vi "GPS -Get Lat Lng from Address.vi"(8 "error in (no error)":errorcluster, 11 "keywords":string="Calgary, Alberta, CANADA") -> (0 "error out":errorcluster, 1 "Lng":dbl, 3 "Lat":dbl, 5 "LngStrg":string, 7 "LatStrg":string)   [LabVIEW 2019]
uses:
  \\mac\Dropbox/gmap.net/GMAP.NET 8.6/data/GMap.NET.Core.dll
  data/GMap.NET.Core.dll
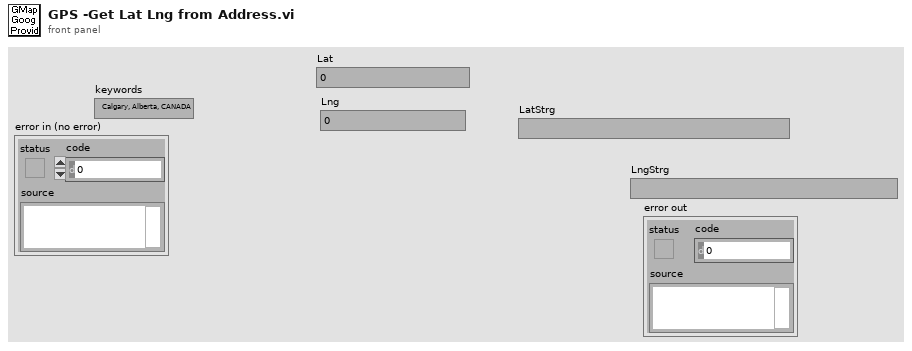
[diagram p1: front panel]
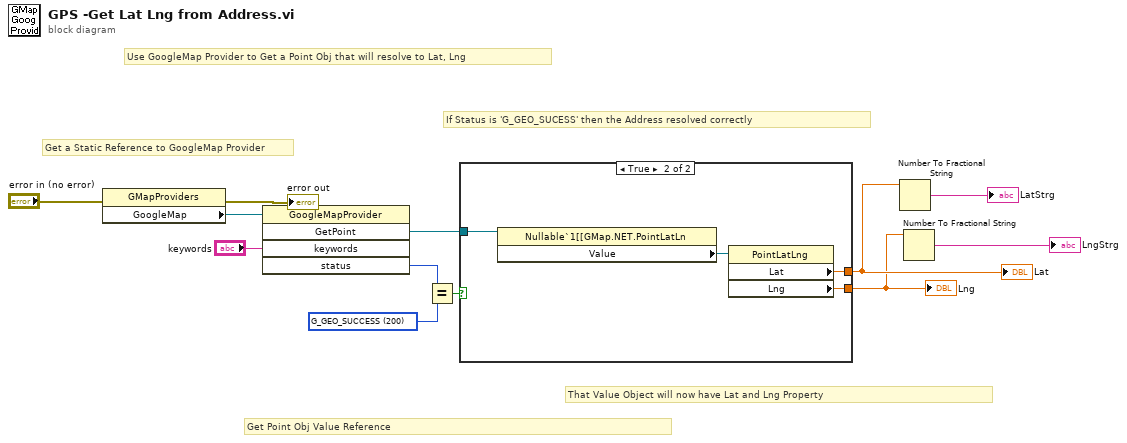
[diagram p0: block diagram]
diagram:
  w9 = 200 items=["G_GEO_SUCCESS"=200, "G_GEO_BAD_REQUEST"=400, "G_GEO_SERVER_ERROR"=500, "G_GEO_MISSING_ADDRESS, G_GEO_MISSING_QUERY"=601, "G_GEO_UNKNOWN_ADDRESS"=602, "G_GEO_UNAVAILABLE_ADDRESS"=603, "G_GEO_UNKNOWN_DIRECTIONS"=604, "G_GEO_BAD_KEY"=610, "G_GEO_TOO_MANY_QUERIES"=620, "ExceptionInCode"=621, "Unknow"=-1] ("status")
  # "That Value Object will now have Lat and Lng Property"
  # "Get Point Obj Value Reference"
  # "If Status is 'G_GEO_SUCESS' then the Address resolved correctly"
  # "Use GoogleMap Provider to Get a Point Obj that will resolve to Lat, Lng"
  # "Get a Static Reference to GoogleMap Provider"
  n1 = property class="GMapProviders"(error in="error in (no error)") -> (error out=→"error out":errorcluster, "GoogleMap"=w12:refnum<k24>)  [unwired: 1 in, 1 out]
  n2 = invoke class="GoogleMapProvider" method="GetPoint"(reference=w12, "keywords"="keywords") -> ("GetPoint"=w11:refnum<k24>, "status"=w10:i32)  [unwired: 3 in, 3 out]
  n3 = Equal?(x=w10, y=w9) -> (x = y?=w8:bool)
  n4 = case shown="True" w8 {
    tunnel: w11 -> [_ w16]
    tunnel: [_ w14] -> w7
    tunnel: [_ w13] -> w6
    frame False {
    }
    frame True {
      n5 = property class="Nullable`1[[GMap.NET.PointLatLn"(reference=w16) -> ("Value"=w15:refnum<k24>)  [unwired: 1 in, 2 out]
      n6 = property class="PointLatLng"(reference=w15) -> ("Lat"=w14:dbl, "Lng"=w13:dbl)  [unwired: 1 in, 2 out]
    }
  }
  "Lng" <- w6
  "Lat" <- w7
  n7 = Number To Fractional String(number=w7) -> (F-format string=→"LatStrg":string)  [unwired: 3 in]
  n8 = Number To Fractional String(number=w6) -> (F-format string=→"LngStrg":string)  [unwired: 3 in]
